vi "SDG60ConfPulse1.vi"(0 "VISA resource name":refnum<visa-resource-name>="USB0::0xF4EC::0x1101::SDG6XEBC5R0119::INSTR", 1 "Amplitude (1.0 Vpp)":dbl=0.1 format="%#.16f", 2 "Offset(1.0 Vpp)":dbl format="%#.16f", 3 "Frequency/Period (1 Hz/s)":dbl=2.0 format="%#.16g", 5 "Channel (1:Channel 1)":i32(ring)=1 items=["Channel 1"=1, "Channel 2"=2], 7 "Freq/Period (T:Freq)":bool, 9 "PulseWidth/Duty(T:PulseWidth)":bool=TRUE, 10 "Delay (s)":dbl format="%#.16f", 11 "error in (no error)":errorcluster, 12 "PulseWidth/Duty (s/%)":dbl=10.0 format="%#.16f", 13 "Rise Edge (s)":dbl format="%#.16f", 14 "Fall Edge (s)":dbl format="%#.16f") -> (4 "VISA resource name out":refnum<visa-resource-name>, 15 "error out":errorcluster)   [LabVIEW 2018]
doc: "Selects the waveform shape, frequency, amplitude, offset, and phase for standard waveforms (including Sine, Square, Ramp, Pulse, DC and Arb).\n\nNotes: \nTo configure other parameters for pulse waveforms please run the Configure Pulse VI. \nTo configure noise waveform please run the Configure Noise VI.\nTo configure other parameters for arbitrary waveforms please run the Create Arbitrary Waveform. \nTo configure PRBS waveform please run the Configure PRBS Waveform VI."
panel:
  out "String":string
  # "Res for both: 6 digits\nAmp: 2mV-20V"
  # "Res for both: 6 digits\nRange: offset -9.999V-Max depends on amplitude, max is however 9.999V"
  # "Range: 1 uHz-200 MHz\nRange: 20 ns-1 Ms\nInternally max res 10 digits for freq, 6 digits for period"
  # "Pulse width range: 3.4 ns-Pulse Period \nDuty Range : 0%-100%\nFor both: 6 digit precision"
  # "Must first set pulse WFM using SDG60ConfSTDWFM\nThen use this vi to change parameters\nIf previous paramaters have been set, may be unable to change them, as generator sets them based off previous settings, may need to initialise to remove previous parameters"
  # "Rise/Fall edge will subtract from pulse width\n11 digit precision\nRange: 2ns-Max dependent on pulsewidth/duty and on other edge"
  # "Range: 0s- Pulse Period\n6 digit precision"
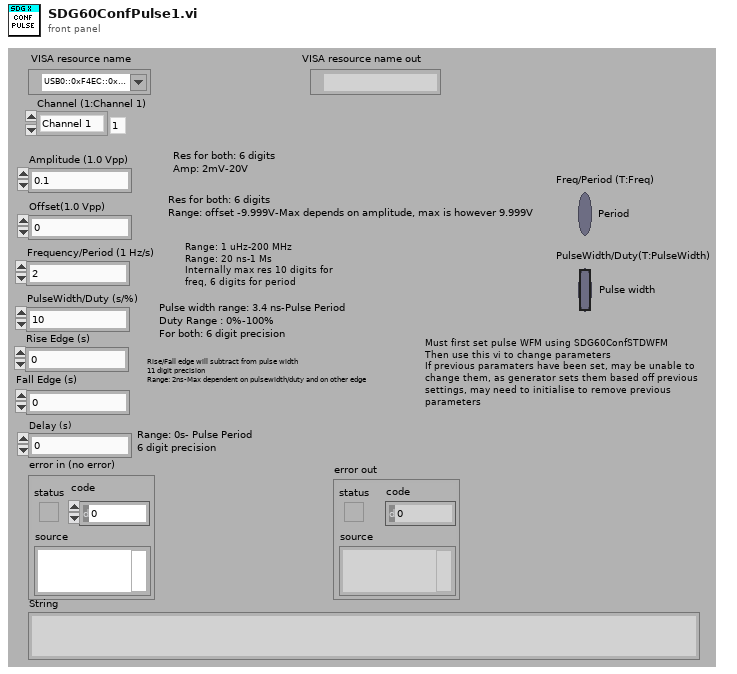
[diagram p1: front panel]
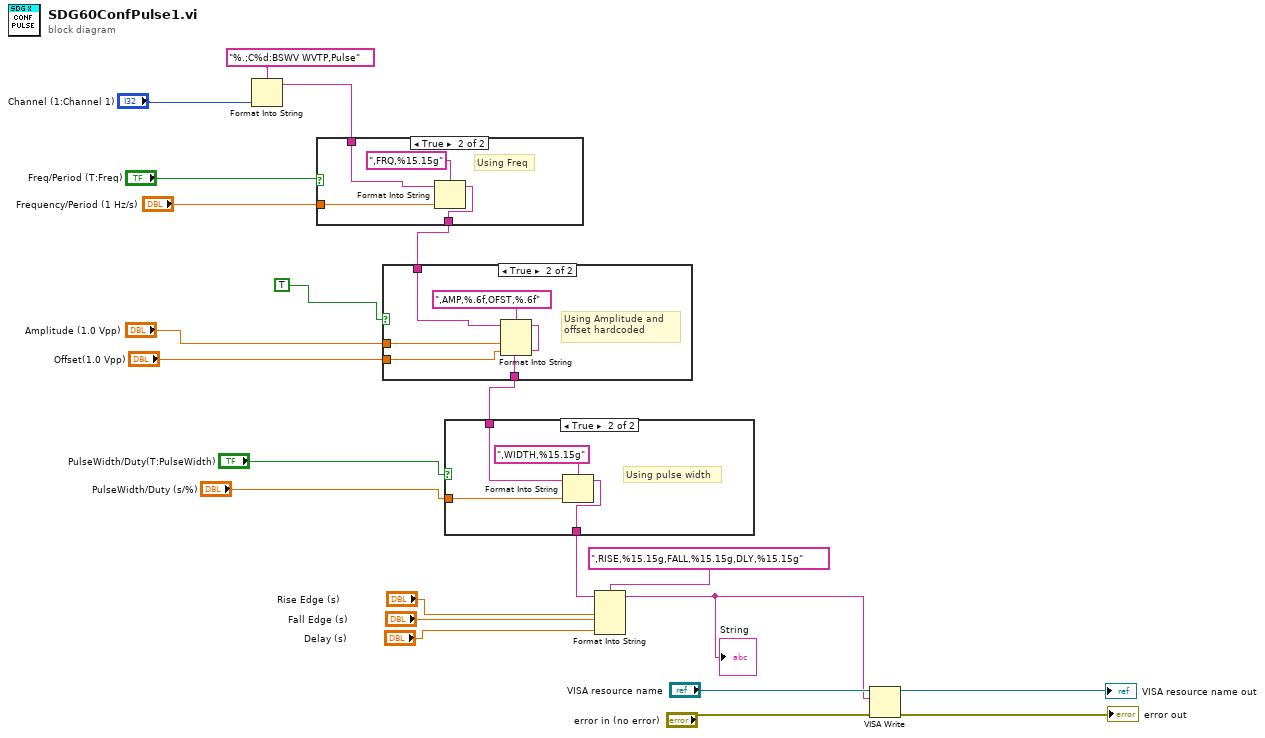
[diagram p0: block diagram]
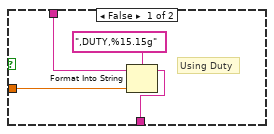
[diagram p2: hidden frame]
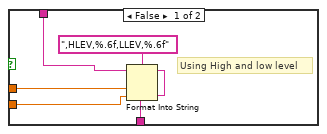
[diagram p3: hidden frame]
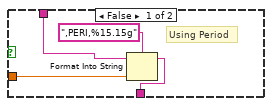
[diagram p4: hidden frame]
diagram:
  n1 = Format Into String(format string="%.;C%d:BSWV WVTP,Pulse", "Channel (1:Channel 1)") -> (resulting string=w16:string)  [unwired: 2 in, 1 out]
  n2 = case shown="True" "Freq/Period (T:Freq)" {
    tunnel: w16 -> [w24 w28]
    tunnel: [w23 w27] -> w13
    tunnel: "Frequency/Period (1 Hz/s)" -> [w25 w29]
    frame False {
      # "Using Period"
      n3 = Format Into String(format string=",PERI,%15.15g", initial string=w24, w25) -> (resulting string=w23:string)  [unwired: 1 in, 1 out]
    }
    frame True {
      # "Using Freq"
      n4 = Format Into String(format string=",FRQ,%15.15g", initial string=w28, w29) -> (resulting string=w27:string)  [unwired: 1 in, 1 out]
    }
  }
  n5 = case shown="True" TRUE {
    tunnel: w13 -> [w33 w38]
    tunnel: [w32 w37] -> w8
    tunnel: "Amplitude (1.0 Vpp)" -> [w34 w39]
    tunnel: "Offset(1.0 Vpp)" -> [w31 w36]
    frame False {
      # "Using High and low level"
      n6 = Format Into String(format string=",HLEV,%.6f,LLEV,%.6f", initial string=w33, w34, w31) -> (resulting string=w32:string)  [unwired: 1 in, 1 out]
    }
    frame True {
      # "Using Amplitude and \noffset hardcoded"
      n7 = Format Into String(format string=",AMP,%.6f,OFST,%.6f", initial string=w38, w39, w36) -> (resulting string=w37:string)  [unwired: 1 in, 1 out]
    }
  }
  n8 = case shown="True" "PulseWidth/Duty(T:PulseWidth)" {
    tunnel: [w42 w46] -> w7
    tunnel: "PulseWidth/Duty (s/%)" -> [w43 w47]
    tunnel: w8 -> [w41 w45]
    frame False {
      # "Using Duty"
      n9 = Format Into String(format string=",DUTY,%15.15g", initial string=w41, w43) -> (resulting string=w42:string)  [unwired: 1 in, 1 out]
    }
    frame True {
      # "Using pulse width"
      n10 = Format Into String(format string=",WIDTH,%15.15g", initial string=w45, w47) -> (resulting string=w46:string)  [unwired: 1 in, 1 out]
    }
  }
  n11 = Format Into String(format string=",RISE,%15.15g,FALL,%15.15g,DLY,%15.15g", initial string=w7, "Rise Edge (s)", "Fall Edge (s)", "Delay (s)") -> (resulting string=w2:string)  [unwired: 1 in, 1 out]
  "String" <- w2
  n12 = VISA Write(VISA resource name="VISA resource name", write buffer=w2, error in (no error)="error in (no error)") -> (VISA resource name out=→"VISA resource name out":refnum<visa-resource-name>, error out=→"error out":errorcluster)  [unwired: 1 out]
